vi "Scale Value (Index).vi"(8 "error in (no error)":errorcluster, 9 "Index":i32, 10 "Value":dbl, 11 "VolatusScaling in":refnum<class "Scaling.lvclass">) -> (0 "error out":errorcluster, 2 "Scaled Value":dbl, 3 "VolatusScaling out":refnum<class "Scaling.lvclass">)   [LabVIEW 2020, in "VolatusData.lvlib" / "Scaling.lvclass"]
uses:
  Scaling.lvclass
  Scaling.lvclass/Scaling.ctl
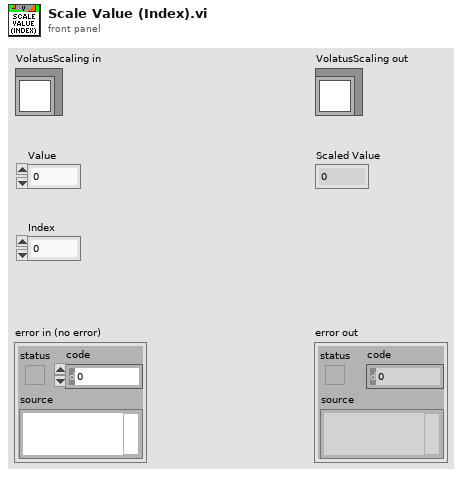
[diagram p1: front panel]
types:
  T1 = typedef "VolatusConfig.lvlib/Scale Type.ctl" = enum16{"None", "Sensor", "Polynomial", "Threshold", "Invert Bool"}
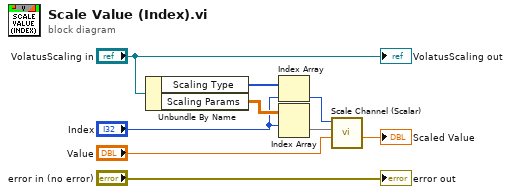
[diagram p0: block diagram]
diagram:
  n1 = Unbundle By Name("VolatusScaling in") -> ("Scaling Type"=w7:T1[], "Scaling Params"=w6:dbl[][])
  n2 = Index Array(array=w7, index="Index") -> (element=w3:T1)
  n3 = Index Array(array=w6, index (row)="Index") -> (element=w4:dbl[])  [unwired: 1 in]
  n4 = call "Scale Channel (Scalar).vi"("Value"="Value", "Scaling Params"=w4, "Scaling Type"=w3) -> ("Scaled Value"=→"Scaled Value":dbl)  [unwired: 8 in]
  "error out" <- "error in (no error)"
  "VolatusScaling out" <- "VolatusScaling in"
